vi "Set Farenheit Mode.vi"(8 "Error In":errorcluster, 10 "Farenheit Mode":bool, 11 "Dual Mode Thermometer in":refnum<class "Dual Mode Thermometer.lvclass">) -> (0 "Error  Out":errorcluster, 3 "Dual Mode Thermometer out":refnum<class "Dual Mode Thermometer.lvclass">)   [LabVIEW 2014, in "Porting from XControls - Dual Mode Thermometer.lvlib" / "Dual Mode Thermometer.lvclass"]
doc: "Copyright (c) 2016 Sze Howe Koh\nThis code is licensed under the MIT license"
uses:
  Dual Mode Thermometer.lvclass
  Dual Mode Thermometer.lvclass/Dual Mode Thermometer.ctl
  src/LabVIEW/LQ Core/Qt/CheckState.ctl
  src/LabVIEW/Qt Widgets/QCheckBox/QCheckBox.lvclass
  src/LabVIEW/LQ Core/Qt/Qt.lvlib
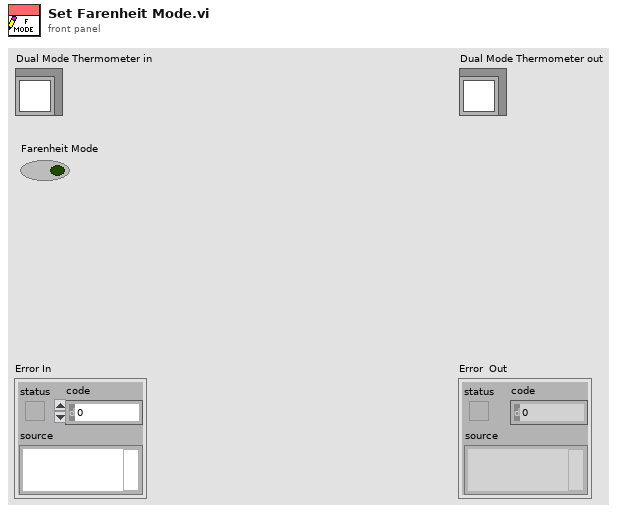
[diagram p1: front panel]
types:
  T1 = typedef "Qt.lvlib/CheckState.ctl" = i32
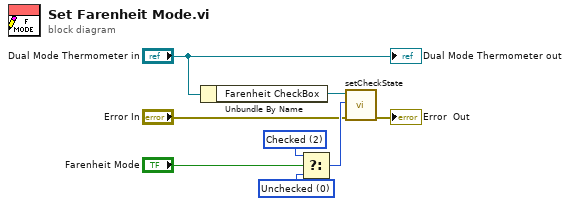
[diagram p0: block diagram]
diagram:
  w4 = T1 0 items=["Unchecked", "PartiallyChecked", "Checked"] ("state")
  w3 = T1 2 items=["Unchecked", "PartiallyChecked", "Checked"] ("state")
  n1 = Unbundle By Name("Dual Mode Thermometer in") -> ("Farenheit CheckBox"=w2:refnum<class "QCheckBox.lvclass">)
  n2 = Select(t=w3, s="Farenheit Mode", f=w4) -> (s? t:f=w6:T1)
  n3 = call "setCheckState.vi"("Error In"="Error In", "state"=w6, "QCheckBox In"=w2) -> ("Error Out"=→"Error  Out":errorcluster)  [unwired: 7 in, 1 out]
  "Dual Mode Thermometer out" <- "Dual Mode Thermometer in"
